vi "Write Reg.vi"(8 "error in (no error)":errorcluster, 10 "Reg":variant, 11 "BCReg in":refnum<class "BCReg.lvclass">) -> (0 "error out":errorcluster, 3 "BCReg out":refnum<class "BCReg.lvclass">)   [LabVIEW 2017, in "BusController.lvlib" / "BCReg.lvclass"]
uses:
  BCReg.lvclass
  BCReg.lvclass/BCReg.ctl
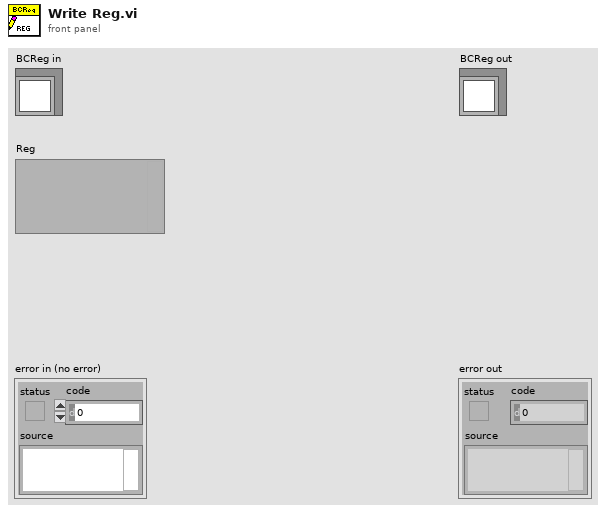
[diagram p1: front panel]
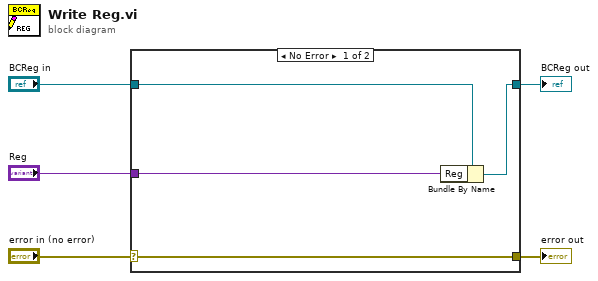
[diagram p0: block diagram]
diagram:
  n1 = case shown="No Error" "error in (no error)" {
    selector: "error in (no error)" -> [w9 w10]
    tunnel: [w9 w10] -> w4
    tunnel: [w7 w11] -> w2
    tunnel: "BCReg in" -> [w8 w11]
    tunnel: "Reg" -> [w6 _]
    frame No Error {
      n2 = Bundle By Name(cluster=w8, "Reg"=w6) -> (w7:refnum<class "BCReg.lvclass">)
    }
    frame Error {
    }
  }
  "error out" <- w4
  "BCReg out" <- w2
